vi "filter.vi"(6 "Threshold":dbl, 10 "Raw1 old":dbl, 11 "Raw1":dbl) -> (3 "Raw1 out":dbl)   [LabVIEW 2017]
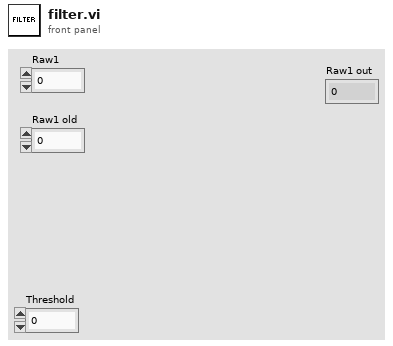
[diagram p1: front panel]
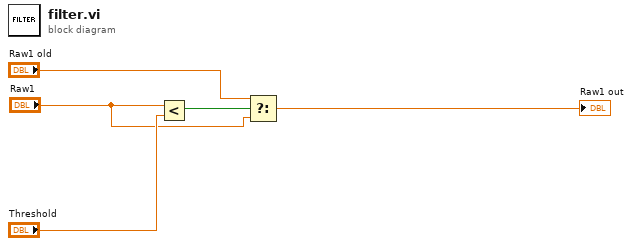
[diagram p0: block diagram]
diagram:
  n1 = Less?(x="Raw1", y="Threshold") -> (x < y?=w4:bool)
  n2 = Select(t="Raw1 old", s=w4, f="Raw1") -> (s? t:f=→"Raw1 out":dbl)
